vi "Mapping.vi"(1 "Min Value":dbl, 2 "Max Value":dbl, 3 "Raw Signal":dbl) -> (0 "Calculated":dbl)   [LabVIEW 2021]
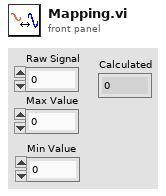
[diagram p1: front panel]
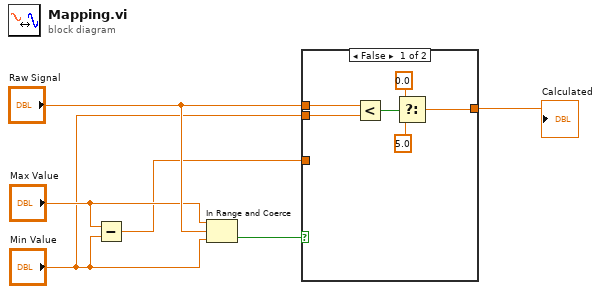
[diagram p0: block diagram]
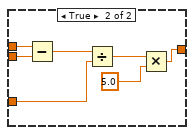
[diagram p2: hidden frame]
diagram:
  n1 = Subtract(x="Max Value", y="Min Value") -> (x-y=w3:dbl)
  n2 = In Range and Coerce(upper limit="Max Value", x="Raw Signal", lower limit="Min Value") -> (In Range?=w6:bool)  [unwired: 1 out]
  n3 = case shown="False" w6 {
    tunnel: "Raw Signal" -> [w12 w16]
    tunnel: w3 -> [_ w15]
    tunnel: "Min Value" -> [w11 w14]
    tunnel: [w7 w13] -> w1
    frame False {
      n4 = Less?(x=w12, y=w11) -> (x < y?=w10:bool)
      n5 = Select(t=0.0, s=w10, f=5.0) -> (s? t:f=w7:dbl)
    }
    frame True {
      n6 = Subtract(x=w16, y=w14) -> (x-y=w19:dbl)
      n7 = Divide(x=w19, y=w15) -> (x/y=w18:dbl)
      n8 = Multiply(x=w18, y=5.0) -> (x*y=w13:dbl)
    }
  }
  "Calculated" <- w1
